vi "Generate Error.vi"(8 "Error In":errorcluster, 10 "Arguments":string[](array[string]), 11 "DEPP Error":T1=enum."Enable") -> (0 "Error Out":errorcluster)   [LabVIEW 2011, in "LVH-Adept.lvlib" / "DEPP.lvlib"]
uses:
  <vilib>/LabVIEW Hacker/Adept/Private/DEPP/DEPP.lvlib
  <vilib>/LabVIEW Hacker/Adept/Private/DEPP/Private/Type Defs/Error.ctl
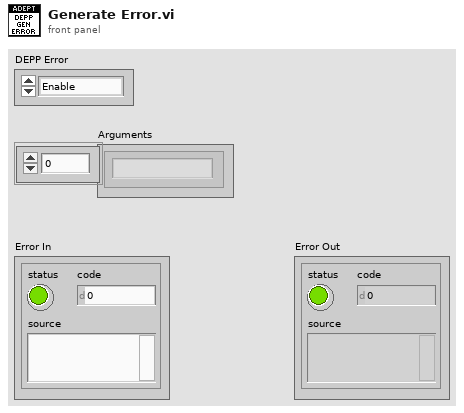
[diagram p1: front panel]
types:
  T1 = typedef "LVH-Adept.lvlib/DEPP.lvlib/Error.ctl" = enum16{"Unknown", "Enable", "Enable Port", "Get Register", "Get Register Repeat", "Get Register Set", "Put Register", "Put Register Repeat", "Put Register Set", "Disable", "Set Pair Size"}
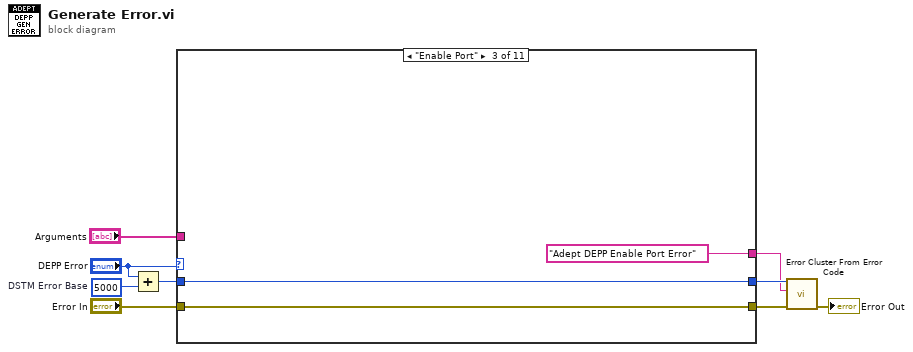
[diagram p0: block diagram]
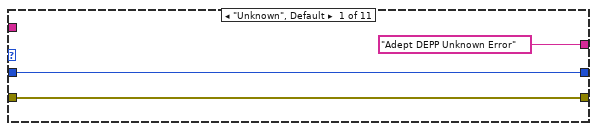
[diagram p2: hidden frame]
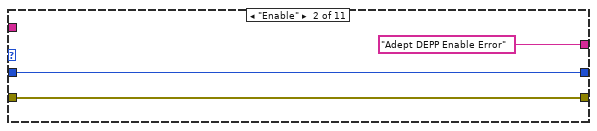
[diagram p3: hidden frame]
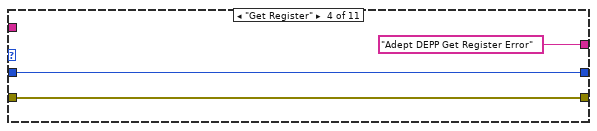
[diagram p4: hidden frame]
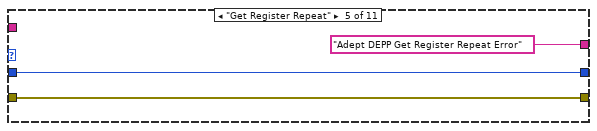
[diagram p5: hidden frame]
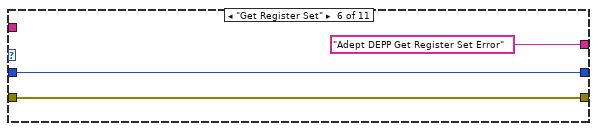
[diagram p6: hidden frame]
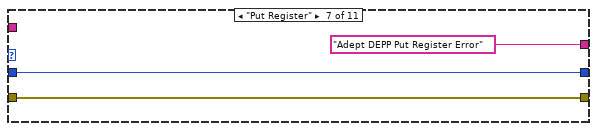
[diagram p7: hidden frame]
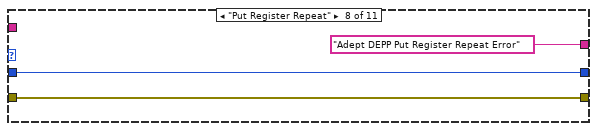
[diagram p8: hidden frame]
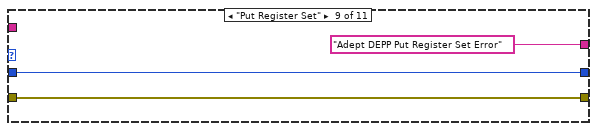
[diagram p9: hidden frame]
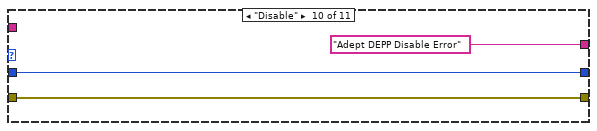
[diagram p10: hidden frame]
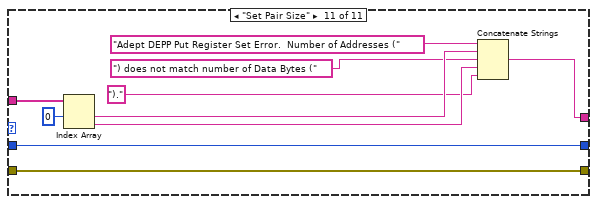
[diagram p11: hidden frame]
diagram:
  w6 = 5000  # DSTM Error Base
  n1 = Add(x="DEPP Error", y=w6) -> (x+y=w3:i32)
  n2 = case shown="\"Enable Port\"" "DEPP Error" {
    tunnel: [w12 w15 w18 w21 w24 w27 w30 w33 w36 w39 w49] -> w8
    tunnel: "Error In" -> [w12 w15 w18 w21 w24 w27 w30 w33 w36 w39 w49]
    tunnel: [w10 w13 w16 w19 w22 w25 w28 w31 w34 w37 w48] -> w5
    tunnel: ["Adept DEPP Unknown Error" "Adept DEPP Enable Error" "Adept DEPP Enable Port Error" "Adept DEPP Get Register Error" "Adept DEPP Get Register Repeat Error" "Adept DEPP Get Register Set Error" "Adept DEPP Put Register Error" "Adept DEPP Put Register Repeat Error" "Adept DEPP Put Register Set Error" "Adept DEPP Disable Error" w40] -> w4
    tunnel: w3 -> [w10 w13 w16 w19 w22 w25 w28 w31 w34 w37 w48]
    tunnel: "Arguments" -> [_ _ _ _ _ _ _ _ _ _ w46]
    frame "Unknown", Default {
    }
    frame "Enable" {
    }
    frame "Enable Port" {
    }
    frame "Get Register" {
    }
    frame "Get Register Repeat" {
    }
    frame "Get Register Set" {
    }
    frame "Put Register" {
    }
    frame "Put Register Repeat" {
    }
    frame "Put Register Set" {
    }
    frame "Disable" {
    }
    frame "Set Pair Size" {
      n3 = Index Array(array=w46, index #1=0 ("index")) -> (element #1=w44:string, element #2=w42:string)  [unwired: 1 in]
      n4 = Concatenate Strings("Adept DEPP Put Register Set Error.  Number of Addresses (", w44, ") does not match number of Data Bytes (", w42, ").") -> (w40:string)
    }
  }
  n5 = call <vilib>:"Error Cluster From Error Code.vi"("error in (no error)"=w8, "error message (\"\")"=w4, "error code (0)"=w5) -> ("error out"=→"Error Out":errorcluster)  [unwired: 6 in]
